vi "Initialise.vi"(8 "error in (no error)":errorcluster, 10 "System In":refnum<class "abs_System.lvclass">, 11 "Node in":refnum<class "abs_Composite.lvclass">) -> (0 "error out":errorcluster, 2 "System Out":refnum<class "abs_System.lvclass">, 3 "Node out":refnum<class "abs_Composite.lvclass">)   [LabVIEW 2021, in "BT.lvlib" / "abs_Composite.lvclass"]
uses:
  abs_Composite.lvclass
  abs_System/abs_System.lvclass
  abs_Composite.lvclass/abs_Composite.ctl
  abs_Node/abs_Node.lvclass
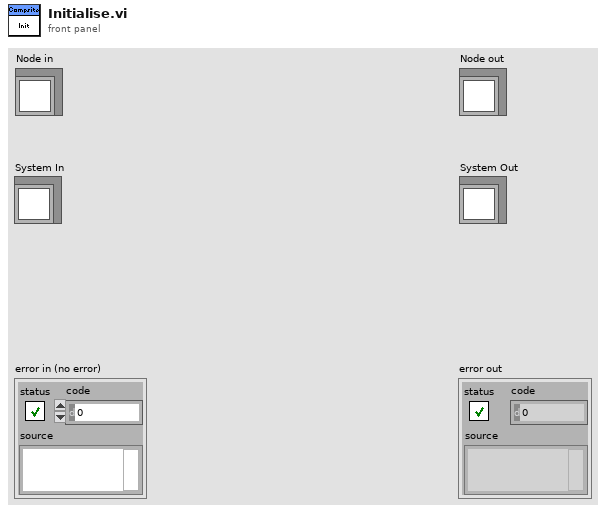
[diagram p1: front panel]
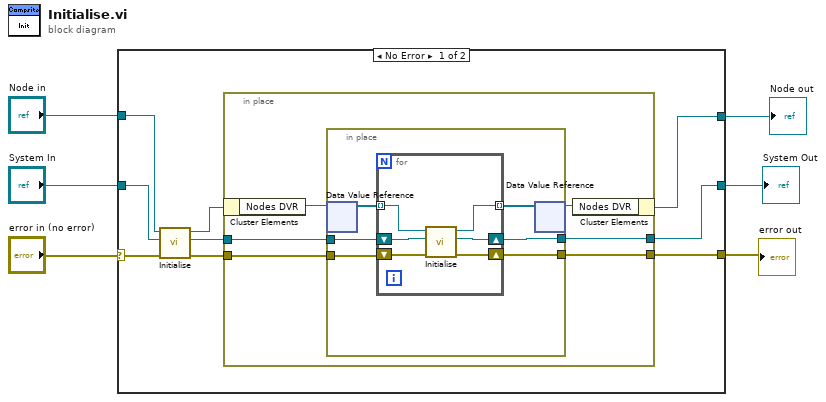
[diagram p0: block diagram]
diagram:
  n1 = case shown="No Error" "error in (no error)" {
    selector: "error in (no error)" -> [w15 w34]
    tunnel: "System In" -> [w14 w35]
    tunnel: "Node in" -> [w13 w36]
    tunnel: [w10 w36] -> w3
    tunnel: [w8 w34] -> w2
    tunnel: [w7 w35] -> w1
    frame No Error {
      n2 = call-parent "Initialise.vi"("error in (no error)"=w15, "System In"=w14, "Node in"=w13) -> ("error out"=w9:errorcluster, "System Out"=w11:refnum<class "abs_System.lvclass">, "Node out"=w12:refnum<class "abs_Composite.lvclass">)  [unwired: 6 in]
      n3 = in-place {
        in-place-border: w11 -> [w20]
        in-place-border: w9 -> [w18]
        in-place-border: [w17] -> w8
        in-place-border: [w16] -> w7
        n4 = in-place-cluster #1(w12) -> ("Nodes DVR"=w21:refnum<data-value>)
        n5 = in-place {
          in-place-border: w20 -> [w26]
          in-place-border: w18 -> [w24]
          in-place-border: [w23] -> w17
          in-place-border: [w22] -> w16
          n6 = in-place-dvr #2(w21) -> (w27:refnum<class "abs_Node.lvclass">[])  [unwired: 1 out]
          n7 = for {
            tunnel: w27 -> [w33] mode=indexing
            tunnel: [w31] -> w25 mode=indexing
            shift-right: [w28] -> w23
            shift-left: w24 -> [w30]
            shift-right: [w29] -> w22
            shift-left: w26 -> [w32]
            n8 = call-dynamic "Initialise.vi"("error in (no error)"=w30, "System In"=w32, "Node in"=w33) -> ("error out"=w28:errorcluster, "System Out"=w29:refnum<class "abs_System.lvclass">, "Node out"=w31:refnum<class "abs_Node.lvclass">)  [unwired: 6 in]
          }
          n9 = in-place-dvr #2(w25) -> (w19:refnum<data-value>)  [unwired: 1 out]
        }
        n10 = in-place-cluster #1("Nodes DVR"=w19) -> (w10:refnum<class "abs_Composite.lvclass">)
      }
    }
    frame Error {
    }
  }
  "error out" <- w2
  "Node out" <- w3
  "System Out" <- w1
